vi "dataUnpackStringArray.vi"(8 "errorIn":errorcluster, 11 "data":variant) -> (0 "errorOut":errorcluster, 3 "StringArray":string[](array[string]))   [LabVIEW 2017]
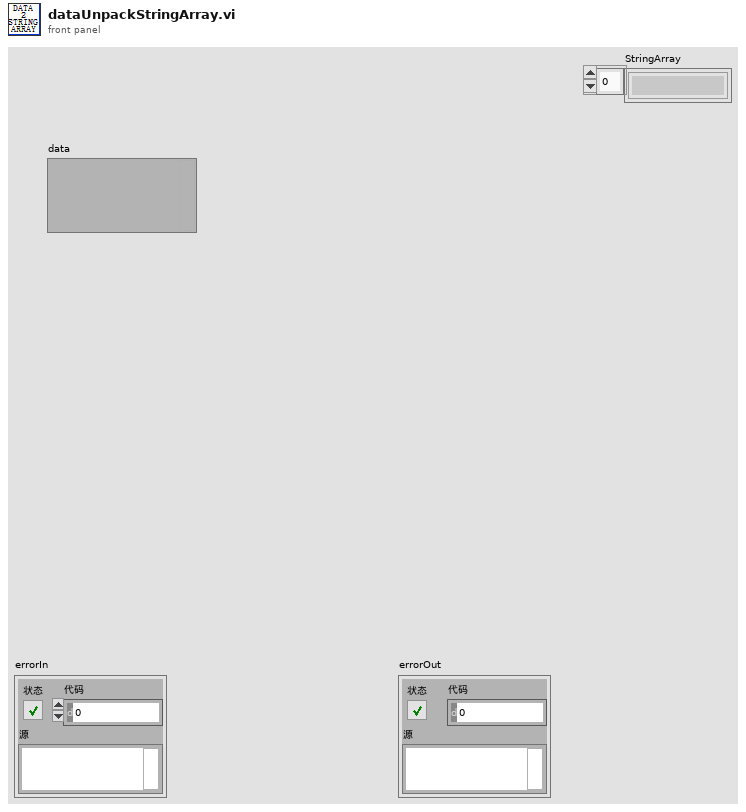
[diagram p1: front panel]
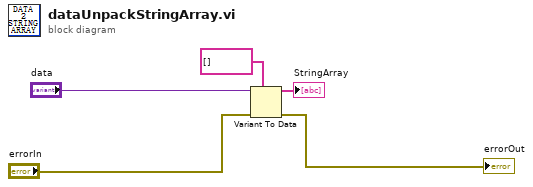
[diagram p0: block diagram]
diagram:
  n1 = Variant To Data(error in="errorIn", type=string[] [], Variant="data") -> (data=→"StringArray":string[], error out=→"errorOut":errorcluster)
